vi "AddTestsFromProjectLibrary.vi"(8 "error in (no error)":errorcluster, 10 "Library":refnum<vi>, 11 "TestSuite in":refnum<class "TestSuite.lvclass">) -> (0 "error out":errorcluster, 3 "TestSuite out":refnum<class "TestSuite.lvclass">)   [LabVIEW 2019, in "TestSuite.lvclass"]
uses:
  TestSuite.lvclass
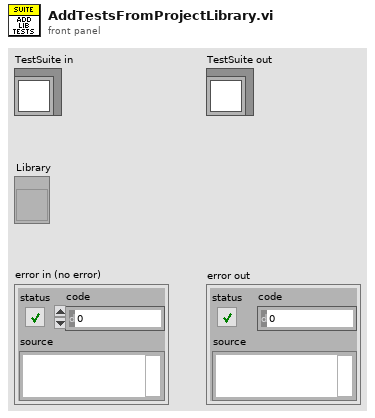
[diagram p1: front panel]
types:
  T1 = enum32{"invalid scope", "public", "private", "protected", "community"}
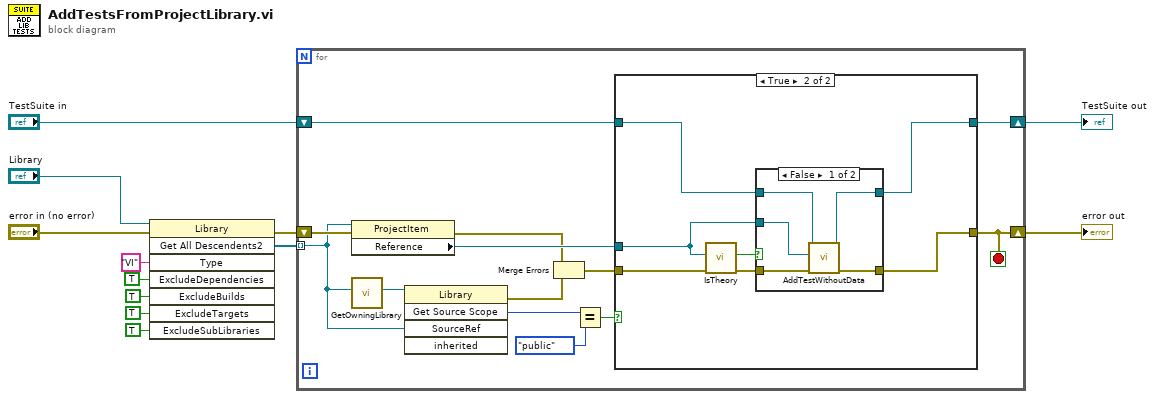
[diagram p0: block diagram]
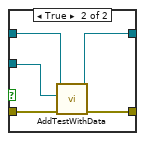
[diagram p3: hidden frame]
diagram:
  n1 = invoke class="Library" method="Get All Descendents2"(reference="Library", error in="error in (no error)", "Type"="VI", "ExcludeDependencies"=TRUE, "ExcludeBuilds"=TRUE, "ExcludeTargets"=TRUE, "ExcludeSubLibraries"=TRUE) -> (error out=w12:errorcluster, "Get All Descendents2"=w11:refnum<vi>[])  [unwired: 1 in, 6 out]
  n2 = for {
    tunnel: w11 -> [w14] mode=indexing
    shift-right: [w20] -> w4
    shift-left: "TestSuite in" -> [w21]
    shift-right: [w16] -> w3
    shift-left: w12 -> [w15]
    stop <- w16 stop-if-true
    n3 = property class="ProjectItem"(reference=w14, error in=w15) -> (error out=w18:errorcluster, "Reference"=w23:refnum<vi>)  [unwired: 1 out]
    n4 = call "GetOwningLibrary.vi"("Parent"=w14) -> ("Owner"=w13:refnum<vi>)  [unwired: 10 in]
    n5 = invoke class="Library" method="Get Source Scope"(reference=w13, "SourceRef"=w14) -> (error out=w17:errorcluster, "GetSourceScope"=w25:T1)  [unwired: 3 in, 3 out]
    n6 = Merge Errors(w18, w17) -> (w19:errorcluster)
    n7 = Equal?(x=w25, y=T1."public") -> (x = y?=w22:bool)
    n8 = case shown="True" w22 {
      tunnel: w23 -> [_ w28]
      tunnel: w21 -> [w27 w31]
      tunnel: [w27 w30] -> w20
      tunnel: w19 -> [w26 w32]
      tunnel: [w26 w29] -> w16
      frame False {
      }
      frame True {
        n9 = call "IsTheory.vi"("error in (no error)"=w32, "VI Refnum"=w28) -> ("error out"=w34:errorcluster, "Is Theory?"=w33:bool)  [unwired: 8 in]
        n10 = case shown="False" w33 {
          tunnel: [w39 w43] -> w29
          tunnel: w31 -> [w38 w41]
          tunnel: [w37 w40] -> w30
          tunnel: w34 -> [w36 w44]
          tunnel: w28 -> [w35 w42]
          frame False {
            n11 = call "AddTestWithoutData.vi"("error in (no error)"=w36, "VI Refnum"=w35, "TestSuite in"=w38) -> ("error out"=w39:errorcluster, "TestSuite out"=w37:refnum<class "TestSuite.lvclass">)  [unwired: 7 in]
          }
          frame True {
            n12 = call "AddTestWithData.vi"("error in (no error)"=w44, "VI Refnum"=w42, "TestSuite in"=w41) -> ("error out"=w43:errorcluster, "TestSuite out"=w40:refnum<class "TestSuite.lvclass">)  [unwired: 7 in]
          }
        }
      }
    }
  }
  "TestSuite out" <- w4
  "error out" <- w3
